vi "Update Attributes In Actor.vi"(6 "Refs":refnum<class "Refs.lvclass">, 7 "Attributes in":refnum<class "Attributes.lvclass">, 9 "Application Ref":refnum<vi>, 10 "Actor Ref":refnum<vi>) -> (5 "Attributes out":refnum<class "Attributes.lvclass">)   [LabVIEW 2025, in "jettl.lvlib"]
uses:
  jettl.lvlib
  Attributes/Attributes.lvclass
  Refs/Refs.lvclass
  Attributes.ctl
  Transport/Transport.lvclass
  Spawn.ctl
  Msg Set.ctl
  Msg/Msg.lvclass
  Actor/Actor.lvclass
  Actor.ctl
  Base Attributes/Base Attributes.lvlib
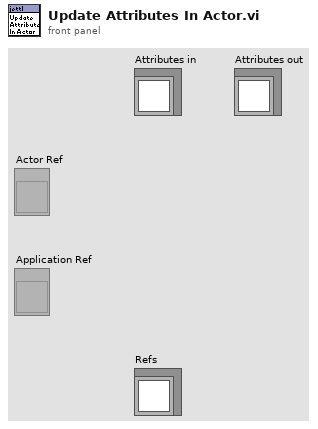
[diagram p1: front panel]
types:
  T1 = typedef "jettl.lvlib/Actor.ctl" = cluster{"Actor Ref":refnum<vi>, "Application Ref":refnum<vi>, "Refs":refnum<class "Refs.lvclass">}
  T2 = typedef "jettl.lvlib/Spawn.ctl" = cluster{"Unified Msg Set":T3, "UID":string, "Parent Attributes":refnum<class "Attributes.lvclass">, "Root":bool, "Persistent Layers":refnum<class "Actor.lvclass">[]}
  T3 = typedef "jettl.lvlib/Msg Set.ctl" = set{refnum<class "Msg.lvclass">}
  T4 = typedef "jettl.lvlib/Attributes.ctl" = cluster{"Spawn":T2, "Actor":T1, "Transport":refnum<class "Transport.lvclass">}
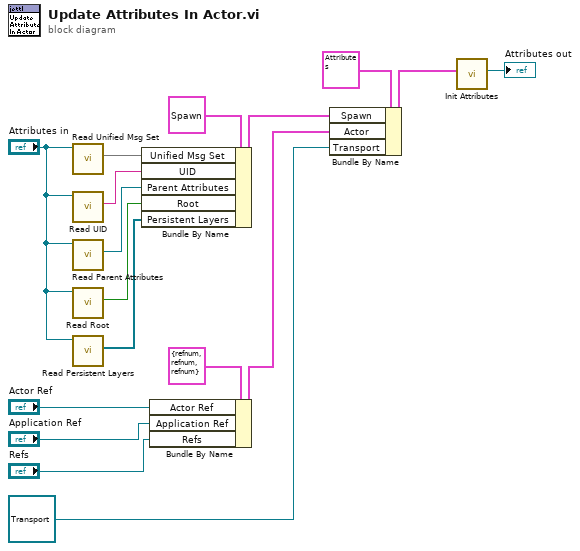
[diagram p0: block diagram]
diagram:
  n1 = call-dynamic "Read Unified Msg Set.vi"("Attributes in"="Attributes in") -> ("Unified Msg Set"=w11:T3)  [unwired: 10 in]
  n2 = call-dynamic "Read UID.vi"("Attributes in"="Attributes in") -> ("UID"=w10:string)  [unwired: 10 in]
  n3 = call-dynamic "Read Parent Attributes.vi"("Attributes in"="Attributes in") -> ("Parent Attributes"=w9:refnum<class "Attributes.lvclass">)  [unwired: 10 in]
  n4 = call-dynamic "Read Root.vi"("Attributes in"="Attributes in") -> ("Root"=w8:bool)  [unwired: 10 in]
  n5 = call-dynamic "Read Persistent Layers.vi"("Attributes in"="Attributes in") -> ("Persistent Layers"=w7:refnum<class "Actor.lvclass">[])  [unwired: 10 in]
  n6 = Bundle By Name(cluster=T2 {"Unified Msg Set"={}, "UID"="", "Parent Attributes"=refnum, "Root"=FALSE, "Persistent Layers"=[]} ("Spawn"), "Unified Msg Set"=w11, "UID"=w10, "Parent Attributes"=w9, "Root"=w8, "Persistent Layers"=w7) -> (w6:T2)
  n7 = Bundle By Name(cluster=T1 {"Actor Ref"=refnum, "Application Ref"=refnum, "Refs"=refnum} ("Actor"), "Actor Ref"="Actor Ref", "Application Ref"="Application Ref", "Refs"="Refs") -> (w4:T1)
  n8 = Bundle By Name(cluster=T4 {"Spawn"={"Unified Msg Set"={}, "UID"="", "Parent Attributes"=refnum, "Root"=FALSE, "Persistent Layers"=[]}, "Actor"={"Actor Ref"=refnum, "Application Ref"=refnum, "Refs"=refnum}, "Transport"=refnum} ("Attributes"), "Spawn"=w6, "Actor"=w4, "Transport"=refnum<class "Transport.lvclass"> refnum ("Actor.Transport")) -> (w14:T4)
  n9 = call "Init Attributes.vi"("Attributes"=w14) -> ("Attributes"=→"Attributes out":refnum<class "Attributes.lvclass">)  [unwired: 10 in]
